vi "SEMAFORO.vi"() -> ()   [LabVIEW 2021]
panel:
  in  "stop":bool
  out "Verde":bool
  out "Amarillo":bool
  out "Rojo":bool
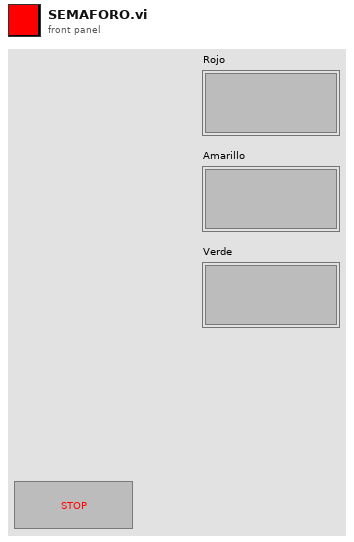
[diagram p1: front panel]
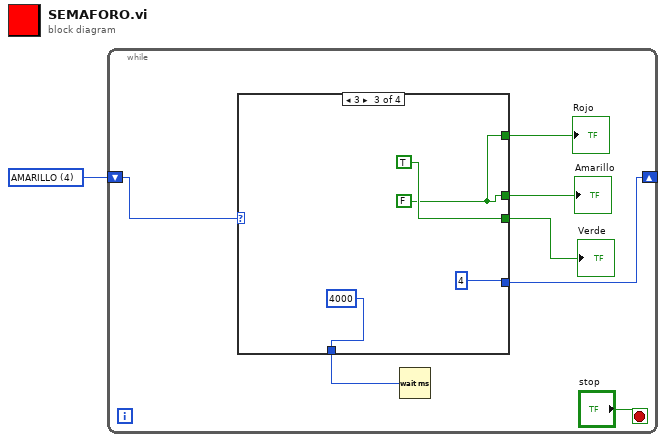
[diagram p0: block diagram]
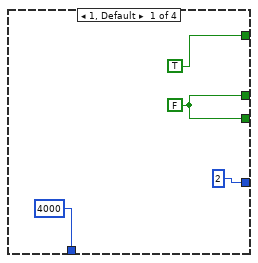
[diagram p2: hidden frame]
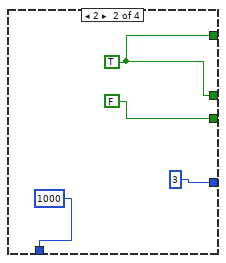
[diagram p3: hidden frame]
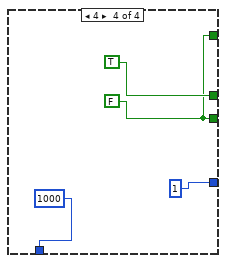
[diagram p4: hidden frame]
diagram:
  w1 = u16 4 items=["ROJO"=1, "ROJO AMARILLO"=2, "VERDE"=3, "AMARILLO"=4, ""=0] ("Text Ring")
  n1 = while {
    shift-right: [w2] -> _
    shift-left: w1 -> [w7]
    stop <- "stop" stop-if-true
    n2 = case shown="3" w7 {
      tunnel: [TRUE w16 w18 w22] -> w6
      tunnel: [w11 w16 w18 TRUE] -> w5
      tunnel: [w11 FALSE TRUE w22] -> w4
      tunnel: [u32 4000 ("milliseconds to wait") 1000 4000 1000] -> w3
      tunnel: [2 3 4 1] -> w2
      frame 1, Default {
        w11 = FALSE
      }
      frame 2 {
        w16 = TRUE
      }
      frame 3 {
        w18 = FALSE
      }
      frame 4 {
        w22 = FALSE
      }
    }
    "Rojo" <- w6
    "Amarillo" <- w5
    "Verde" <- w4
    n3 = Wait (ms)(milliseconds to wait=w3) -> ()  [unwired: 1 out]
  }
